vi "Initialize.vi"(8 "error in (no error)":errorcluster, 11 "VLC Wrapper in":refnum<class "VLC Wrapper.lvclass">) -> (0 "error out":errorcluster, 3 "VLC Wrapper out":refnum<class "VLC Wrapper.lvclass">)   [LabVIEW 2020, in "VLC Wrapper.lvclass"]
doc: "This is a factory method that will encapsulate all complexity needed to start sending the console commands. Initially the required steps you must set the Application Name and the Working directory parameters. If you do not set those values, the Application Name will be empty and the working directory will be C:. It will also pass the command \"dir\" wihtout any options."
uses:
  VLC Wrapper.lvclass
  C:/Users/fflores/Documents/GitHub Projects/LabVIEW-CLI-Wrapper/Console Wrapper/Console Wrapper.lvclass
  Console Wrapper/Console Wrapper.lvclass/Console Wrapper.ctl
  Console Wrapper/Write Application Name.vi
  Console Wrapper/Write Working Directory.vi
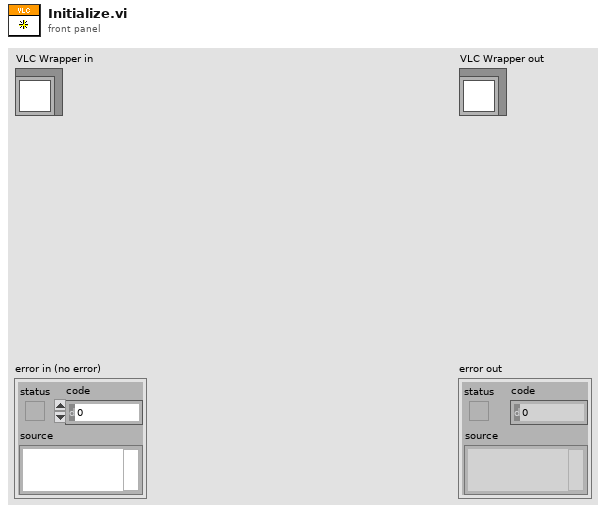
[diagram p1: front panel]
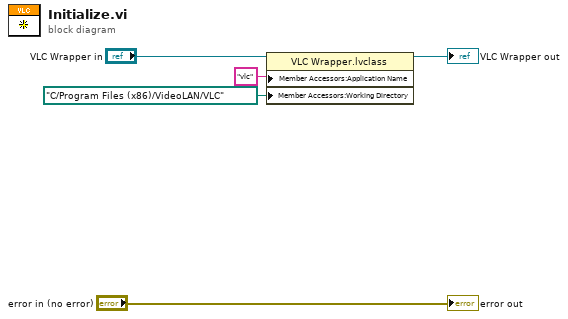
[diagram p0: block diagram]
diagram:
  n1 = property class="VLC Wrapper.lvclass"(reference="VLC Wrapper in", "Member Accessors:Application Name"="vlc" ("Application Name"), "Member Accessors:Working Directory"=path "C:/Program Files (x86)/VideoLAN/VLC" ("Working Directory")) -> (reference out=→"VLC Wrapper out":refnum<class "VLC Wrapper.lvclass">)  [unwired: 1 in, 1 out]
  "error out" <- "error in (no error)"
